vi "ReaderCore.vi"(1 "Initiational":bool caption="Initiational (internal)", 2 "Close":bool caption="Close (internal)", 3 "Filename":string caption="Filename (internal)", 8 "NXT":T1={"Hardware"="NXT", "Flattened String"=""}) -> (11 "NXT":T1={"Hardware"="NXT", "Flattened String"=""})   [LabVIEW 2010, in "Packet Recorder.lvlib"]
uses:
  Packet Recorder.lvlib
  <vilib>/NXT/Subs/LVHSConnector.ctl
  Remote Interface/Remote Interface.lvlib
panel:
  out "EOF":bool
  out "Button Data":string
  out "Joystick Data":string
  out "total time":u32
  out "Stored Filename":string
  in  "stored loop index":u32
  out "initial ms time":u32
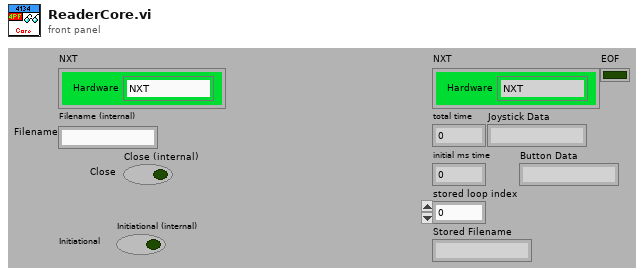
[diagram p1: front panel]
types:
  T1 = typedef "LVHSConnector.ctl" = cluster{"Hardware":string, "Flattened String":string}
  T2 = enum16{"Selected Joysticks", "Selected Buttons", "Selected Buttons and Joysticks", "Custom Call (w/ Aux. Data)"}
  T3 = cluster{"1B1-12:2B1-12:1POV:2POV":bool[], "1LXY:RXY:2LXY:RXY":bool[]}
  T4 = typedef "FTC ControllerState.ctl" = cluster{"Left X":i8, "Left Y":i8, "Right X":i8, "Right Y":i8, "Button Encoding 9-12":u8, "Button Encoding 1-8":u8, "POV":T5}
  T5 = typedef "FTC POVState.ctl" = i8
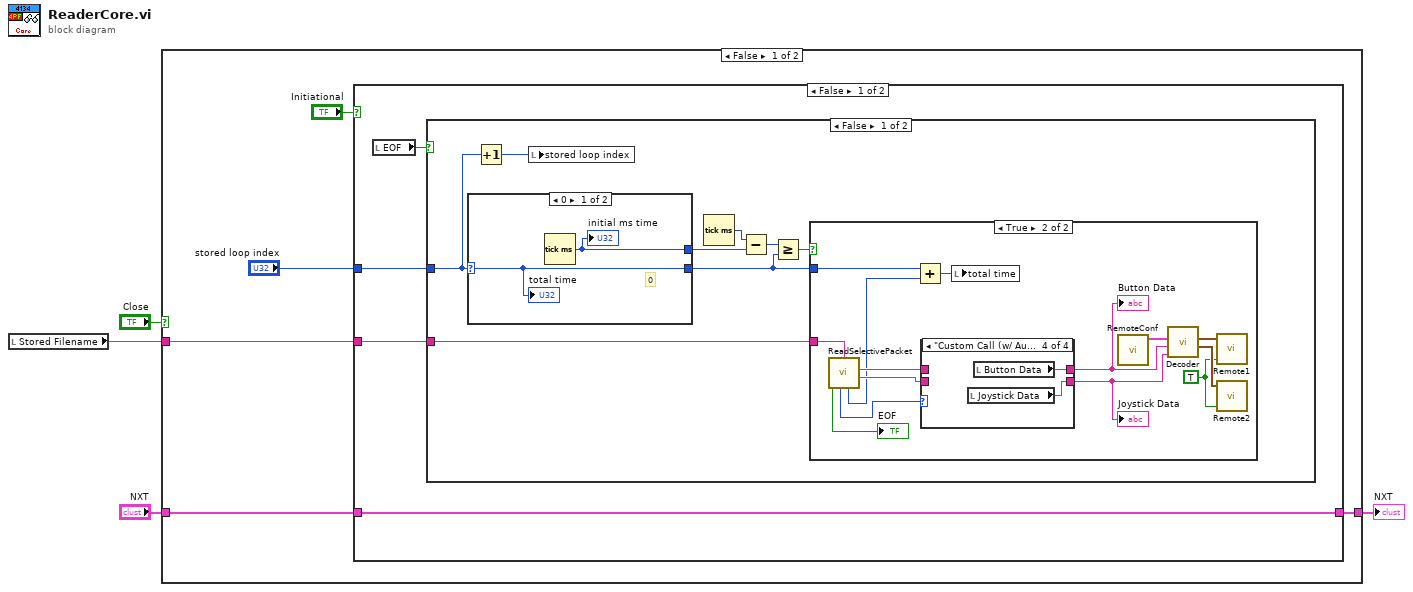
[diagram p0: block diagram]
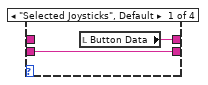
[diagram p3: hidden frame]
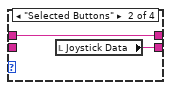
[diagram p4: hidden frame]
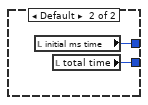
[diagram p6: hidden frame]
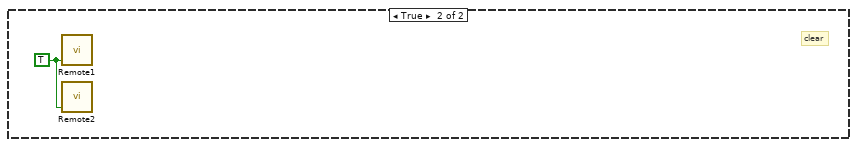
[diagram p7: hidden frame]
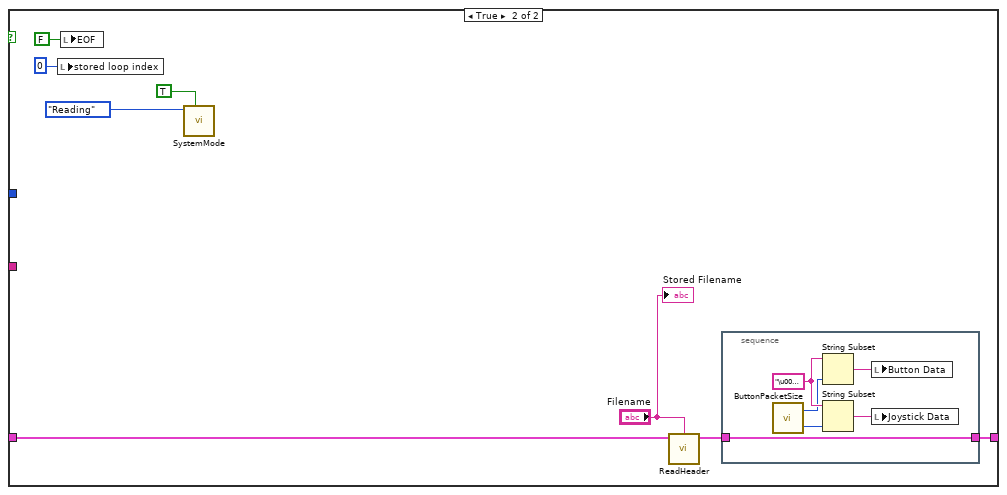
[diagram p8: hidden frame]
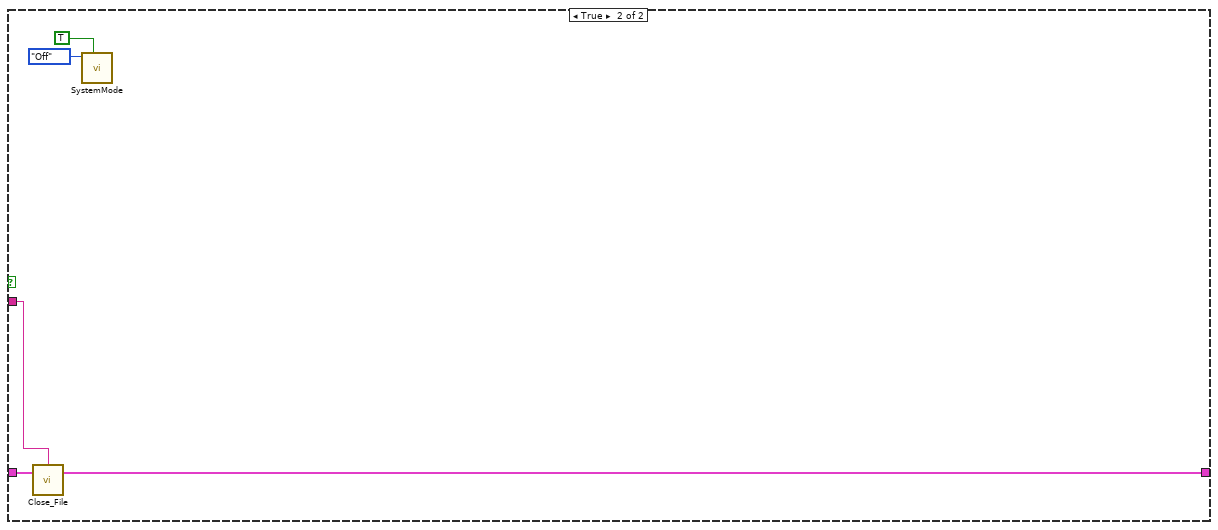
[diagram p9: hidden frame]
diagram:
  n1 = local read "Stored Filename"() -> (w3:string)
  n2 = case shown="False" "Close" {
    tunnel: "NXT" -> [w8 w66]
    tunnel: w3 -> [w7 w67]
    tunnel: [w5 w65] -> w2
    frame False {
      n3 = case shown="False" "Initiational" {
        tunnel: w7 -> [w12 _]
        tunnel: w8 -> [w11 w56]
        tunnel: "stored loop index" -> [w13 _]
        tunnel: [w11 w49] -> w5
        frame False {
          n4 = local read "EOF"() -> (w10:bool)
          n5 = case shown="False" w10 {
            tunnel: w13 -> [w18 _]
            tunnel: w12 -> [w17 _]
            frame False {
              n6 = case shown="0" w18 {
                selector: w18 -> [w44 _]
                tunnel: [w45 w47] -> w20
                tunnel: [w44 w46] -> w15
                frame 0 {
                  # "0"
                  n7 = Tick Count (ms)() -> (millisecond timer value=w45:u32)
                  "initial ms time" <- w45
                  "total time" <- w44
                }
                frame Default {
                  n8 = local read "initial ms time"() -> (w47:u32)
                  n9 = local read "total time"() -> (w46:u32)
                }
              }
              n10 = Increment(x=w18) -> (x+1=w21:u32)
              n11 = local write "stored loop index"(w21) -> ()
              n12 = Tick Count (ms)() -> (millisecond timer value=w19:u32)
              n13 = Subtract(x=w19, y=w20) -> (x-y=w16:u32)
              n14 = Greater Or Equal?(x=w16, y=w15) -> (x >= y?=w14:bool)
              n15 = case shown="True" w14 {
                tunnel: w17 -> [_ w35]
                tunnel: w15 -> [_ w24]
                frame False {
                }
                frame True {
                  w28 = TRUE ("Write?")
                  n16 = call "ReadSelectivePacket.vi"("Filename"=w35) -> ("Button Data"=w31:string, "Joystick Data"=w32:string, "Time (MS)"=w23:u32, "Packet Type"=w34:T2, "EOF"=→"EOF":bool)  [unwired: 3 in, 2 out]
                  n17 = Add(x=w24, y=w23) -> (x+y=w27:u32)
                  n18 = case shown="\"Custom Call (w/ Aux. Data)\"" w34 {
                    tunnel: w32 -> [w36 _ w41 _]
                    tunnel: w31 -> [_ w38 w40 _]
                    tunnel: [w36 w39 w41 w42] -> w26
                    tunnel: [w37 w38 w40 w43] -> w25
                    frame "Selected Joysticks", Default {
                      n19 = local read "Button Data"() -> (w37:string)
                    }
                    frame "Selected Buttons" {
                      n20 = local read "Joystick Data"() -> (w39:string)
                    }
                    frame "Selected Buttons and Joysticks" {
                    }
                    frame "Custom Call (w/ Aux. Data)" {
                      n21 = local read "Joystick Data"() -> (w42:string)
                      n22 = local read "Button Data"() -> (w43:string)
                    }
                  }
                  "Joystick Data" <- w26
                  "Button Data" <- w25
                  n23 = local write "total time"(w27) -> ()
                  n24 = call "RemoteConf.vi"() -> ("Conf"=w33:T3)  [unwired: 11 in]
                  n25 = call "Decoder.vi"("Joystick Data"=w26, "Button Data"=w25, "Conf"=w33) -> ("Controller 2 State"=w29:T4, "Controller 1 State"=w30:T4)  [unwired: 7 in]
                  n26 = call "Remote1.vi"("Write?"=w28, "Write Controller State"=w30) -> ()  [unwired: 2 in, 1 out]
                  n27 = call "Remote2.vi"("Write?"=w28, "Write Controller State"=w29) -> ()  [unwired: 2 in, 1 out]
                }
              }
            }
            frame True {
              w48 = TRUE ("Write?")
              # "clear"
              n28 = call "Remote1.vi"("Write?"=w48) -> ()  [unwired: 3 in, 1 out]
              n29 = call "Remote2.vi"("Write?"=w48) -> ()  [unwired: 3 in, 1 out]
            }
          }
        }
        frame True {
          n30 = local write "stored loop index"(u32 0 ("stored loop index")) -> ()
          n31 = local write "EOF"(FALSE ("EOF")) -> ()
          n32 = call "SystemMode.vi"("Write?"=TRUE, "ModeInput"=enum16{"Off", "Reading", "Writing"}."Reading") -> ()  [unwired: 9 in, 1 out]
          n33 = call "ReadHeader.vi"("Filename"="Filename", "NXT"=w56) -> ("NXT"=w50:T1)  [unwired: 7 in]
          n34 = stacked-sequence {
            tunnel: w50 -> [w57]
            tunnel: [w57] -> w49
            frame #0 {
              w62 = "\u0000\u0000\u0000\u0000\u0000\u0000\u0000\u0000" ("concatenated string")
              n35 = call "ButtonPacketSize.vi"() -> ("joystick packet size"=w60:u8, "button packet size"=w61:u8)  [unwired: 2 in]
              n36 = String Subset(string=w62, length (rest)=w61) -> (substring=w58:string)  [unwired: 1 in]
              n37 = String Subset(string=w62, length (rest)=w60) -> (substring=w59:string)  [unwired: 1 in]
              n38 = local write "Button Data"(w58) -> ()
              n39 = local write "Joystick Data"(w59) -> ()
            }
          }
          "Stored Filename" <- "Filename"
        }
      }
    }
    frame True {
      n40 = call <vilib>:"Close_File.vi"("NXT"=w66, "Filename"=w67) -> ("NXT"=w65:T1)  [unwired: 2 in]
      n41 = call "SystemMode.vi"("Write?"=TRUE, "ModeInput"=enum16{"Off", "Reading", "Writing"}."Off") -> ()  [unwired: 9 in, 1 out]
    }
  }
  "NXT" <- w2
